vi "update_waypoints.vi"(11 "Mission in":refnum<class "Mission.lvclass">) -> (3 "Mission out":refnum<class "Mission.lvclass">)   [LabVIEW 2011, in "Mission.lvclass"]
uses:
  Mission.lvclass
  Mission.lvclass/Mission.ctl
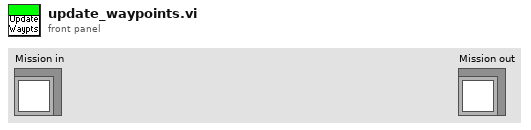
[diagram p1: front panel]
types:
  T1 = enum16{"Round Buoy", "Drive", "Pass Buoys", "Station Keeping"}
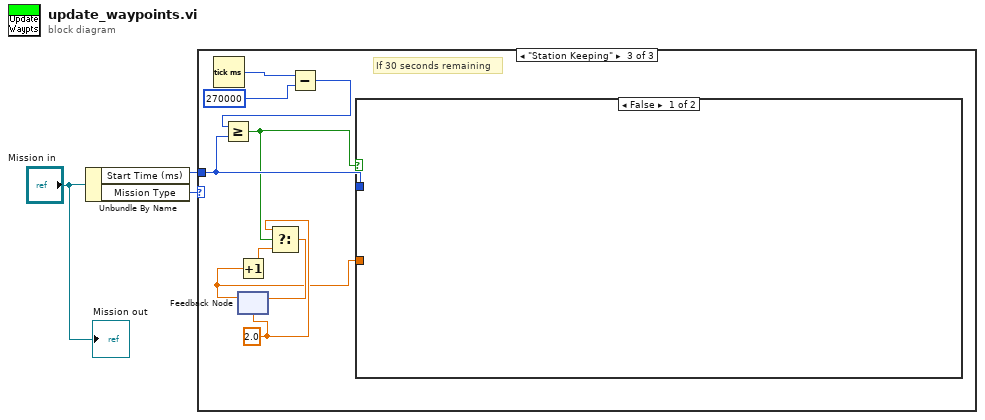
[diagram p0: block diagram]
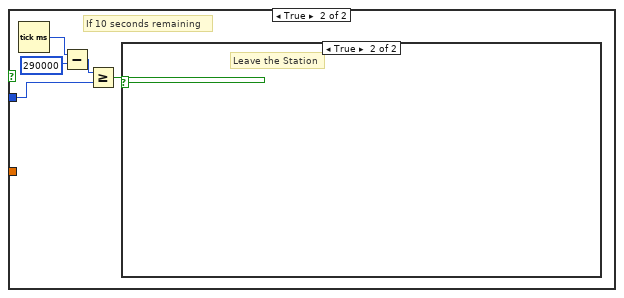
[diagram p4: hidden frame]
diagram:
  n1 = Unbundle By Name("Mission in") -> ("Start Time (ms)"=w1:u32, "Mission Type"=w3:T1)
  n2 = case shown="\"Station Keeping\"" w3 {
    tunnel: w1 -> [_ _ w10]
    frame "Round Buoy", Default {
    }
    frame "Pass Buoys" {
    }
    frame "Station Keeping" {
      w6 = 2.0
      # "If 30 seconds remaining"
      n3 = Tick Count (ms)() -> (millisecond timer value=w12:u32)
      n4 = feedback #1(w6) -> (w4:dbl)
      n5 = Increment(x=w4) -> (x+1=w7:dbl)
      n6 = Subtract(x=w12, y=u32 270000) -> (x-y=w9:u32)
      n7 = Greater Or Equal?(x=w9, y=w10) -> (x >= y?=w8:bool)
      n8 = Select(t=w6, s=w8, f=w7) -> (s? t:f=w5:dbl)
      n9 = feedback-in #1(w5) -> ()
      n10 = case shown="False" w8 {
        tunnel: w10 -> [_ w14]
        tunnel: w4 -> [_ _]
        frame False {
        }
        frame True {
          # "If 10 seconds remaining"
          n11 = Tick Count (ms)() -> (millisecond timer value=w17:u32)
          n12 = Subtract(x=w17, y=u32 290000) -> (x-y=w15:u32)
          n13 = Greater Or Equal?(x=w15, y=w14) -> (x >= y?=w13:bool)
          n14 = case shown="True" w13 {
            frame False {
              # "Ride a wall"
            }
            frame True {
              # "Leave the Station"
            }
          }
        }
      }
    }
  }
  "Mission out" <- "Mission in"
